vi "GUItoPLCInt.vi"(10 "Real Input Array":i32[](array[numeric])) -> (2 "DB Output Array":u8[](array[numeric]))   [LabVIEW 2023]
panel:
  out "Array":bool[](array[boolean])
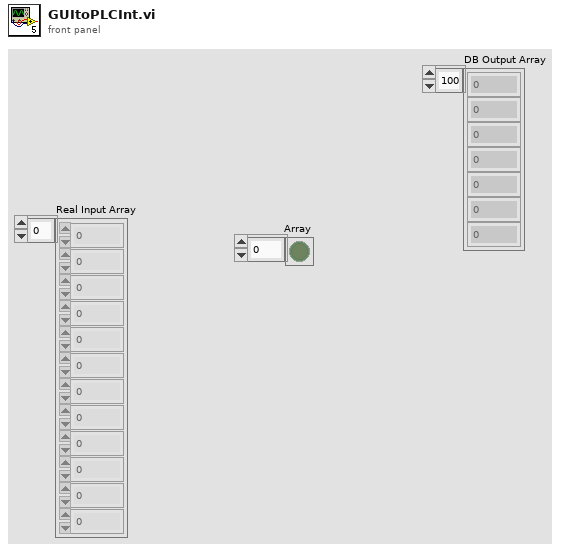
[diagram p1: front panel]
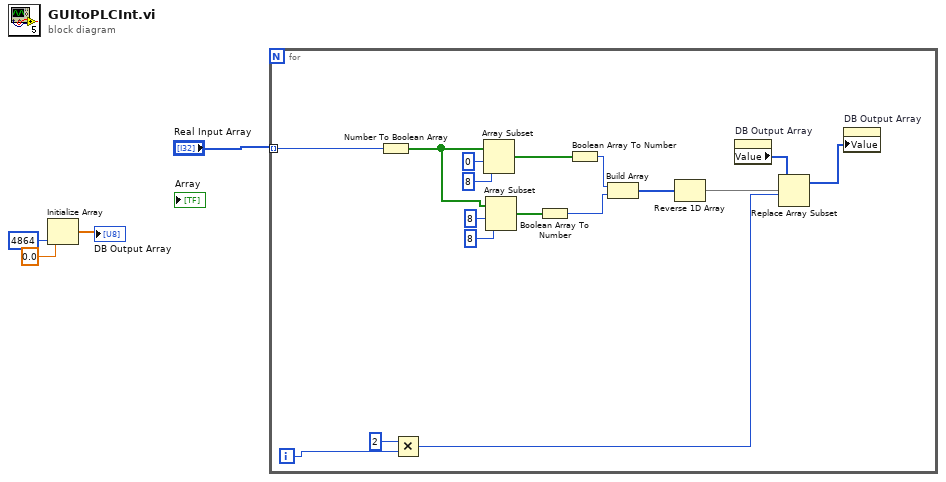
[diagram p0: block diagram]
diagram:
  n1 = Initialize Array(0.0 ("element"), 4864 ("dimension size")) -> (→"DB Output Array":dbl[])
  n2 = for {
    tunnel: "Real Input Array" -> [w5] mode=indexing
    i -> [w12]
    n3 = Number To Boolean Array(number=w5) -> (Boolean array=w17:bool[])
    n4 = Multiply(x=2, y=w12) -> (x*y=w11:i32)
    n5 = Array Subset(array=w17, index=0, length=8) -> (w7:bool[])
    n6 = Array Subset(array=w17, index=8, length=8) -> (w6:bool[])
    n7 = Boolean Array To Number(Boolean array=w6) -> (number=w15:u32)
    n8 = Boolean Array To Number(Boolean array=w7) -> (number=w16:u32)
    n9 = Build Array(w16, w15) -> (w9:u32[])
    n10 = Reverse 1D Array(array=w9) -> (reversed array=w8:u32[])
    n11 = property on="DB Output Array" class="Arr (strict)"() -> ("Value"=w14:u8[])  [unwired: 2 in, 2 out]
    n12 = Replace Array Subset(array=w14, new element=w8, index=w11) -> (w13:u8[])
    n13 = property on="DB Output Array" class="Arr (strict)"("Value"=w13) -> ()  [unwired: 2 in, 2 out]
  }
